vi "ZCAN_FilterAck.vi"(0 "error in (no error)":errorcluster caption="错误输入（无错误）", 2 "can_index_handle":u32, 5 "can_index":u32) -> (14 "error out":errorcluster caption="错误输出", 15 "启动滤波成功？":bool, 16 "can_index_handle(out)":u32, 19 "can_index(out)":u32)   [LabVIEW 2018]
doc: "启动滤波"
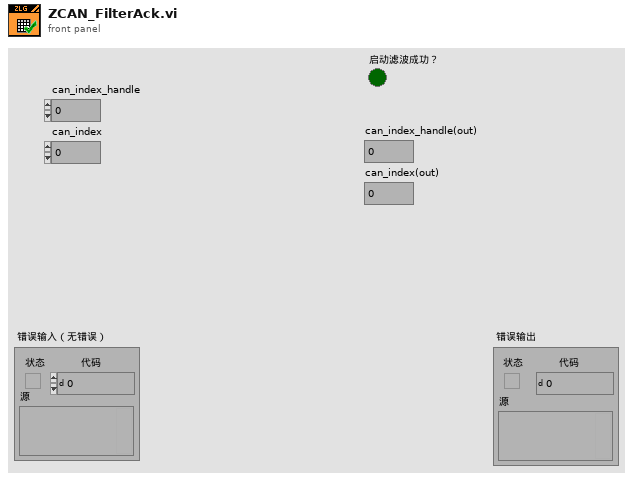
[diagram p1: front panel]
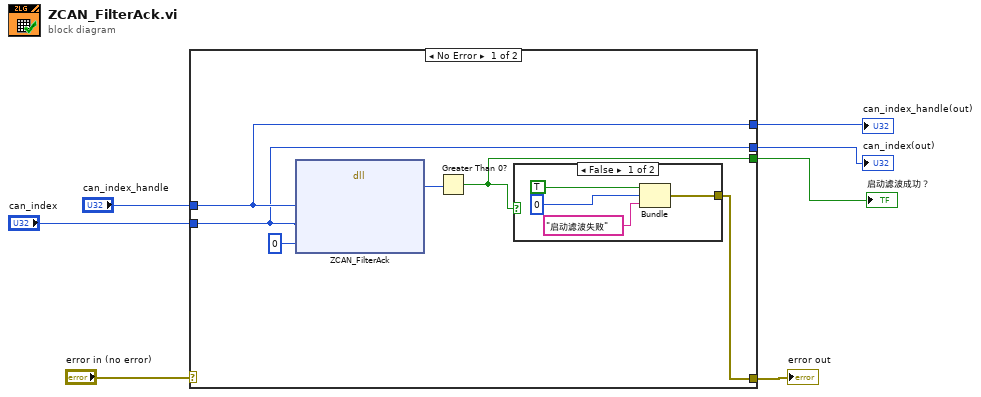
[diagram p0: block diagram]
diagram:
  n1 = case shown="No Error" "error in (no error)" {
    selector: "error in (no error)" -> [_ w18]
    tunnel: [w13 w18] -> w6
    tunnel: "can_index_handle" -> [w11 _]
    tunnel: "can_index" -> [w10 _]
    tunnel: [w11 _] -> w3
    tunnel: [w10 _] -> w2
    tunnel: [w8 _] -> w1
    frame No Error {
      n2 = dll-call lib="PTH2zabs CUsersadminDesktop\"2020版本 zlgcan_labview_20220510 zlgcan_demo_PCIECANFD-400U_mergebinzlgcan_wrap.dll" fn="ZCAN_FilterAck"("device_handle"=w11, "can_index"=w10, "ack"=0 ("clear")) -> ("return"=w9:u32)  [unwired: 6 in, 2 out]
      n3 = Greater Than 0?(x=w9) -> (x > 0?=w8:bool)
      n4 = case shown="False" w8 {
        tunnel: [w14 _] -> w13
        frame False {
          n5 = Bundle("status"=TRUE, "code"=0, "消息"="启动滤波失败") -> (w14:cluster{"status":bool, "code":i32, "消息":string})  [unwired: 1 in]
        }
        frame True {
        }
      }
    }
    frame Error {
    }
  }
  "error out" <- w6
  "can_index_handle(out)" <- w3
  "can_index(out)" <- w2
  "启动滤波成功？" <- w1
